vi "get_file_data.vi"() -> (1 "名称":string, 2 "数组":dbl[][](array[numeric]))   [LabVIEW 2014]
panel:
  out "拆分的路径":path
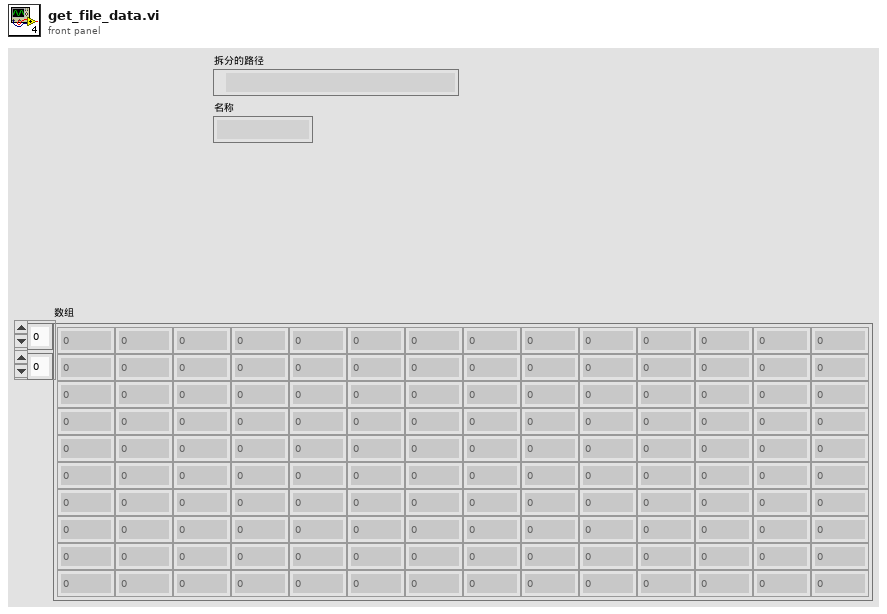
[diagram p1: front panel]
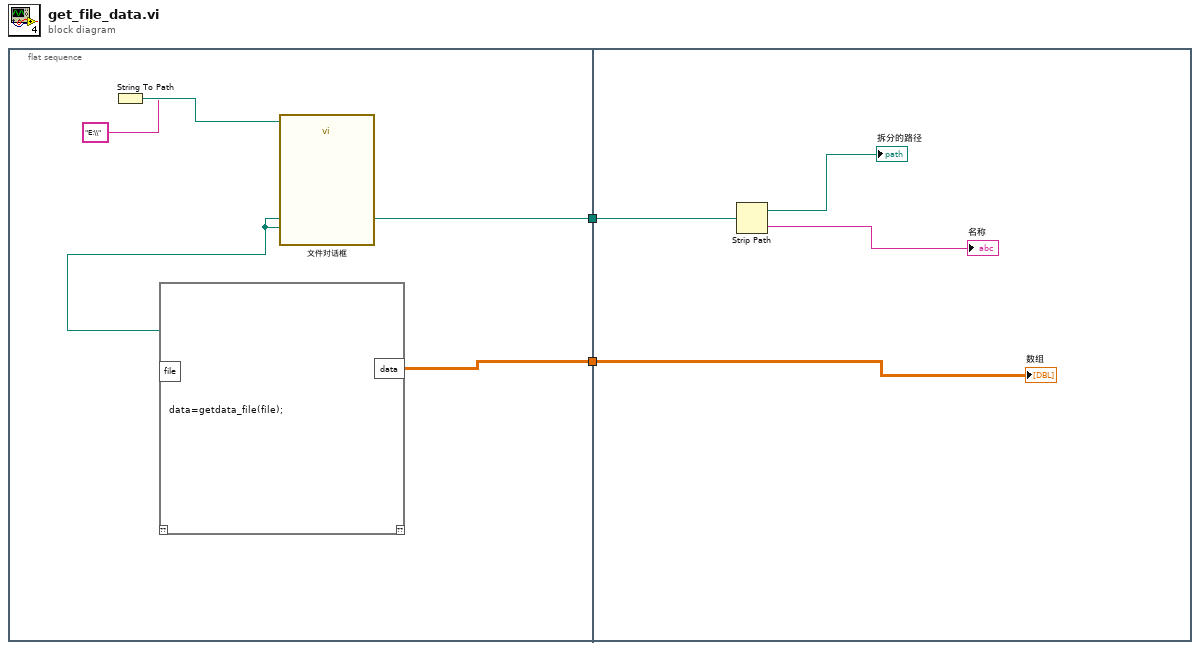
[diagram p0: block diagram]
diagram:
  n1 = flat-sequence {
    tunnel: [w6] -> w2
    tunnel: [w3] -> w1
    tunnel: w2 -> [w10]
    tunnel: w1 -> [w9]
    frame #0 {
      n2 = String To Path(string="E:\\") -> (path=w5:path)
      n3 = call "文件对话框"("start path"=w5) -> ("selected path"=w3:path)  [unwired: 11 in, 3 out]
      n4 = script code="data=getdata_file(file);"("file"=w3) -> ("data"=w6:cdb[][])  [unwired: 1 in, 1 out]
    }
    frame #1 {
      n5 = Strip Path(path=w9) -> (stripped path=→"拆分的路径":path, name=→"名称":string)
      "数组" <- w10
    }
  }
